vi "Run query.vi"(0 "InfluxDB in":refnum<class "InfluxDB Client.lvclass">, 5 "Database name":string, 7 "Query":string, 9 "Precision (ms)":T1=enum."milliseconds", 11 "error in (no error)":errorcluster) -> (4 "InfluxDB out":refnum<class "InfluxDB Client.lvclass">, 6 "JSON data":string, 15 "error out":errorcluster)   [LabVIEW 2015, in "InfluxDB Client.lvclass"]
doc: "Runs a query on a specific database and returns the result as JSON data."
uses:
  InfluxDB Client.lvclass
  Time precision.ctl
  InfluxDB Client.lvclass/InfluxDB Client.ctl
  <vilib>/httpClient/LabVIEWHTTPClient.lvlib
panel:
  out "Status":string
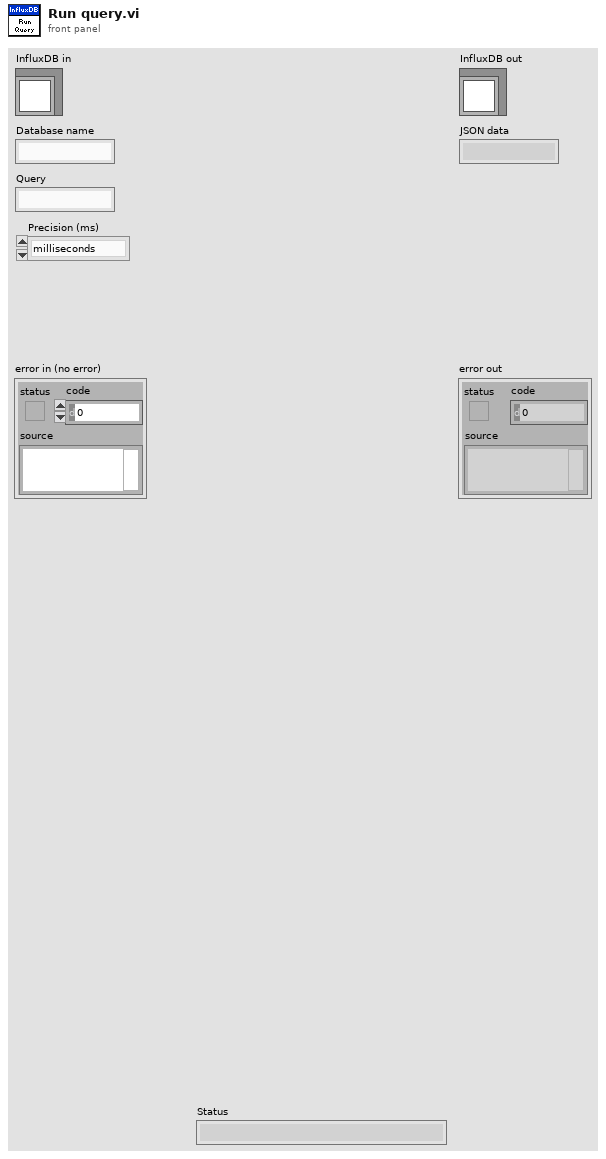
[diagram p1: front panel]
types:
  T1 = typedef "InfluxDB Client.lvclass/Time precision.ctl" = enum16{"seconds", "milliseconds", "microseconds"}
  T2 = typedef "LabVIEWHTTPClient.lvlib/ClientHandle.ctl" = refnum<k1>
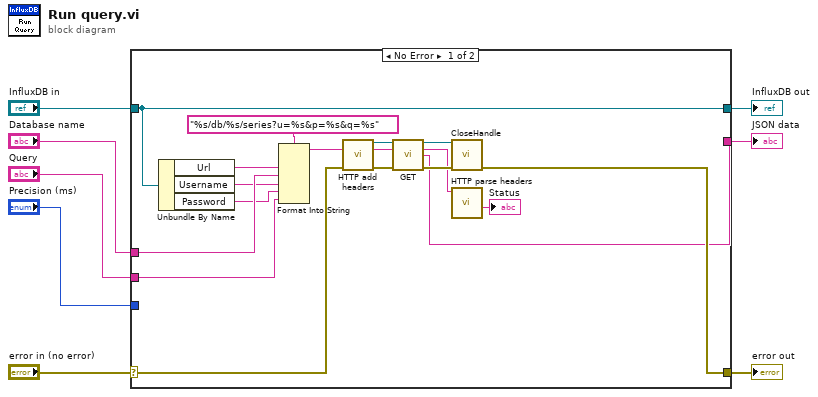
[diagram p0: block diagram]
diagram:
  n1 = case shown="No Error" "error in (no error)" {
    selector: "error in (no error)" -> [w11 w27]
    tunnel: [w19 w27] -> w7
    tunnel: [w25 w26] -> w5
    tunnel: "InfluxDB in" -> [w25 w26]
    tunnel: [w12 _] -> w2
    tunnel: "Database name" -> [w16 _]
    tunnel: "Query" -> [w13 _]
    tunnel: "Precision (ms)" -> [_ _]
    frame No Error {
      n2 = Unbundle By Name(w25) -> ("Url"=w23:string, "Username"=w15:string, "Password"=w14:string)
      n3 = Format Into String(format string="%s/db/%s/series?u=%s&p=%s&q=%s" ("url"), w23, w16, w15, w14, w13) -> (resulting string=w20:string)  [unwired: 2 in, 1 out]
      n4 = call "HTTP add headers.vi"("error in (no error)"=w11) -> ("client handle out"=w10:T2, "error out"=w9:errorcluster)  [unwired: 13 in]
      n5 = call <vilib>:"GET.vi"("client handle"=w10, "url"=w20, "error in (no error)"=w9) -> ("client handle out"=w22:T2, "headers"=w18:string, "body"=w12:string, "error out"=w21:errorcluster)  [unwired: 9 in]
      n6 = call <vilib>:"CloseHandle.vi"("client handle"=w22, "error in (no error)"=w21) -> ("error out"=w19:errorcluster)  [unwired: 13 in]
      n7 = call "HTTP parse headers.vi"("HTTP headers"=w18) -> ("Status"=→"Status":string)  [unwired: 8 in, 2 out]
    }
    frame Error {
    }
  }
  "error out" <- w7
  "InfluxDB out" <- w5
  "JSON data" <- w2
